vi "GetTerms4.vi"(0 "XRef":T11, 1 "State In":T10) -> (14 "Terms":T2, 15 "Fatal Error Out":T1)   [LabVIEW 2015, in "Set Object Parameters.xnode"]
uses:
  Set Object Parameters.xnode
  <vilib>/XNodeSupport/XNodeXNodeRef.ctl
  State.ctl
  <vilib>/XNodeSupport/XNodeTerm4Array.ctl
  <vilib>/XNodeSupport/XNodeTerm4.ctl
  <vilib>/XNodeSupport/XNodeString.ctl
  <vilib>/XNodeSupport/XNodeVariant.ctl
  <vilib>/XNodeSupport/XNodeRect32.ctl
  <vilib>/XNodeSupport/XNodeInt.ctl
  <vilib>/XNodeSupport/XNodeBool.ctl
  <vilib>/XNodeSupport/XNodeTermDirection.ctl
  <vilib>/XNodeSupport/XNodeErrorCluster.ctl
  JSON Object.lvclass
  JSON Datatype/JSON Null.lvclass
  JSON String/JSON String.lvclass
  JSON Numeric/JSON Numeric.lvclass
  JSON Boolean/JSON Boolean.lvclass
  JSON Array/JSON Array.lvclass
  dimensions.vi
  <vilib>/XNodeSupport/NI_XNodeSupport.lvlib
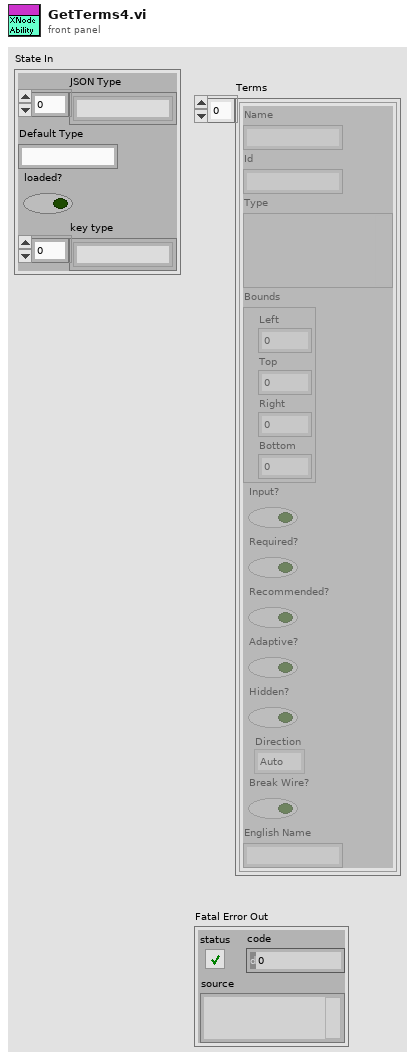
[diagram p1: front panel]
types:
  T1 = typedef "NI_XNodeSupport.lvlib/XNodeErrorCluster.ctl" = errorcluster
  T2 = typedef "NI_XNodeSupport.lvlib/XNodeTerm4Array.ctl" = T3[]
  T3 = typedef "NI_XNodeSupport.lvlib/XNodeTerm4.ctl" = cluster{"Name":T4, "Id":T4, "Type":T5, "Bounds":T6, "Input?":T8, "Required?":T8, "Recommended?":T8, "Adaptive?":T8, "Hidden?":T8, "Direction":T9, "Break Wire?":T8, "English Name":T4}
  T4 = typedef "NI_XNodeSupport.lvlib/XNodeString.ctl" = string
  T5 = typedef "NI_XNodeSupport.lvlib/XNodeVariant.ctl" = variant
  T6 = typedef "NI_XNodeSupport.lvlib/XNodeRect32.ctl" = cluster{"Left":T7, "Top":T7, "Right":T7, "Bottom":T7}
  T7 = typedef "NI_XNodeSupport.lvlib/XNodeInt.ctl" = i32
  T8 = typedef "NI_XNodeSupport.lvlib/XNodeBool.ctl" = bool
  T9 = typedef "NI_XNodeSupport.lvlib/XNodeTermDirection.ctl" = enum32{"Auto", "Up", "Down", "Left", "Right", "Center"}
  T10 = typedef "Set Object Parameters.xnode/State.ctl" = cluster{"JSON Type":string[], "Default Type":string, "loaded?":bool, "key type":string[]}
  T11 = typedef "NI_XNodeSupport.lvlib/XNodeXNodeRef.ctl" = refnum<vi>
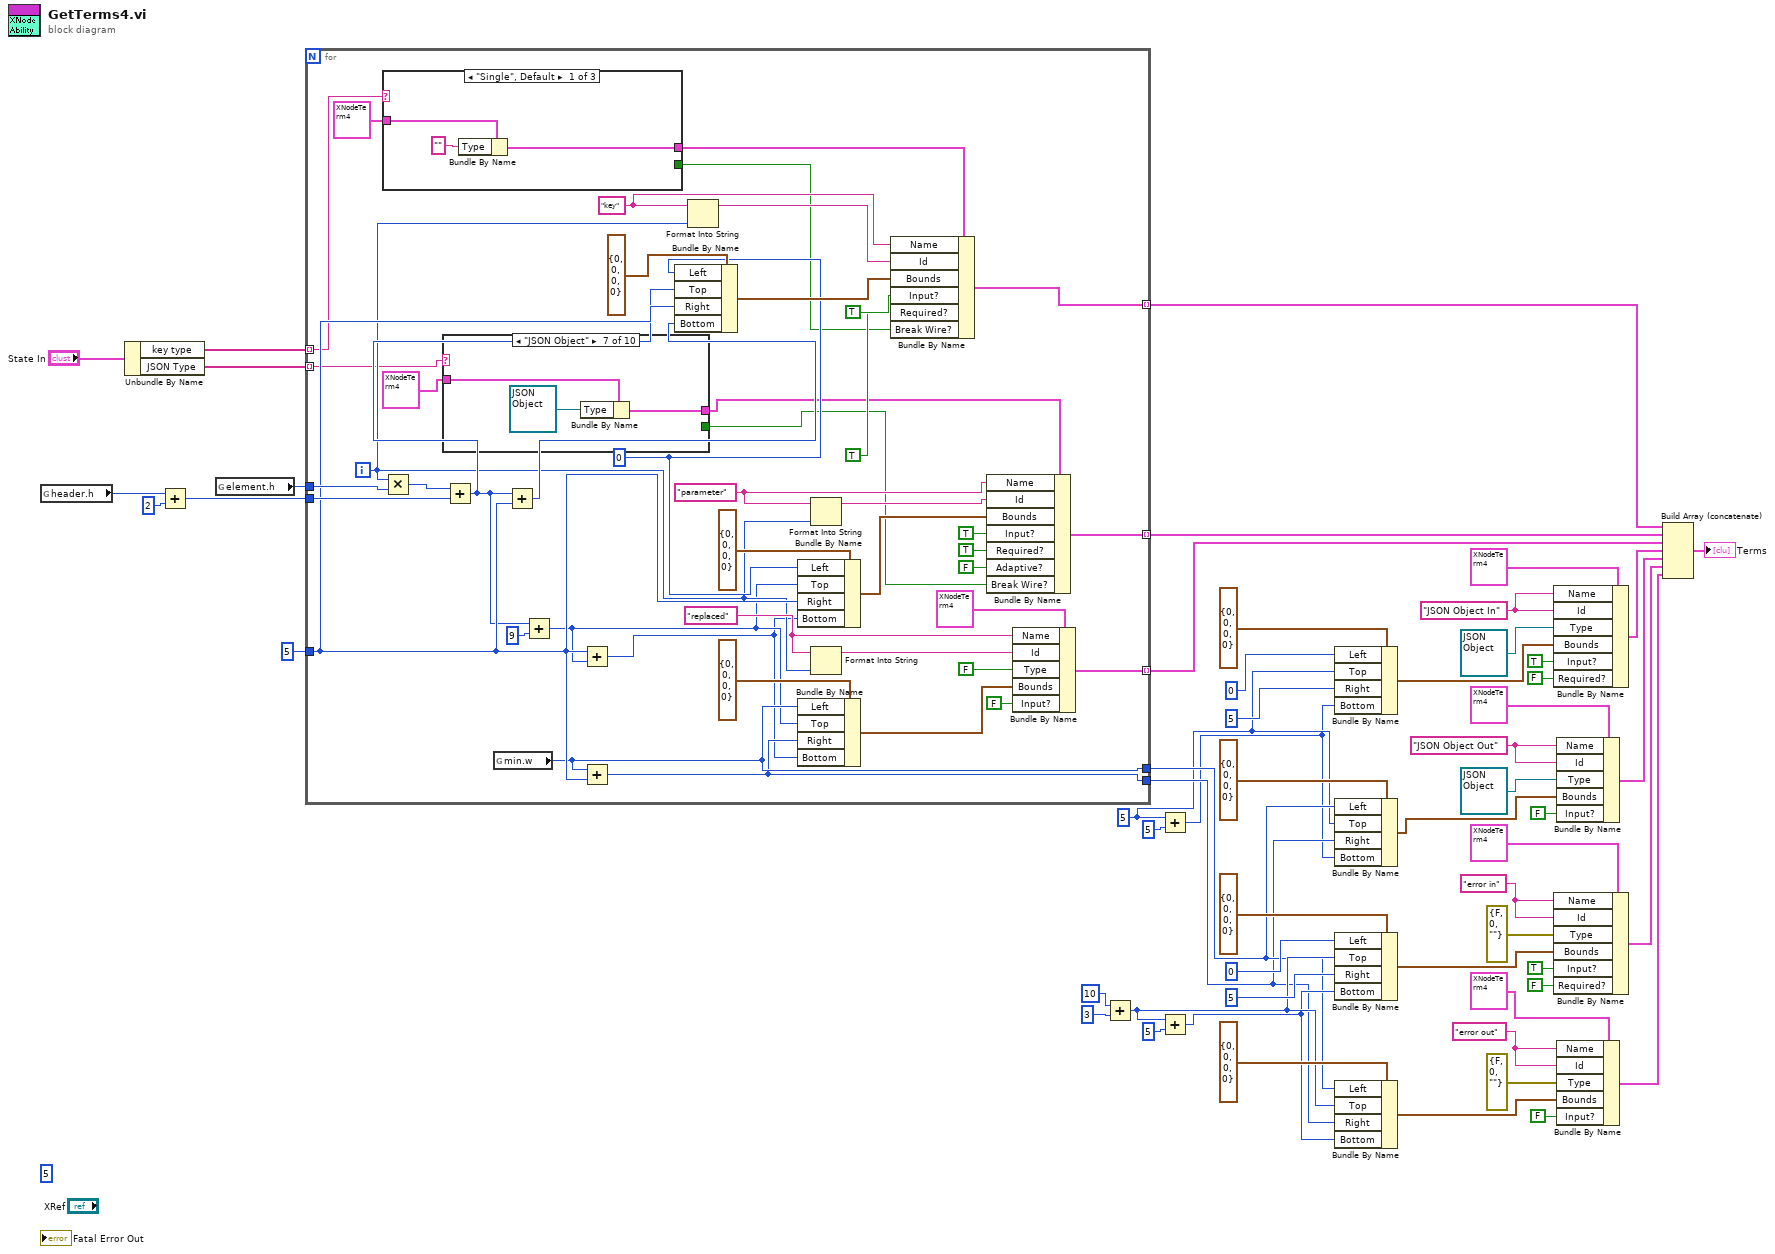
[diagram p0: block diagram]
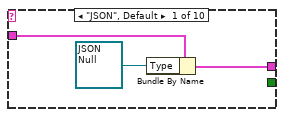
[diagram p2: hidden frame]
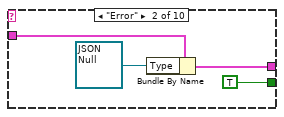
[diagram p3: hidden frame]
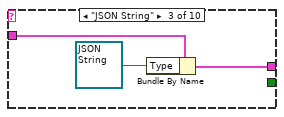
[diagram p4: hidden frame]
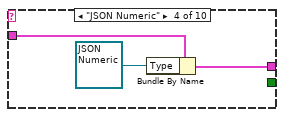
[diagram p5: hidden frame]
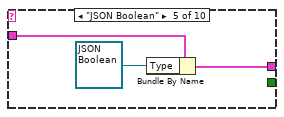
[diagram p6: hidden frame]
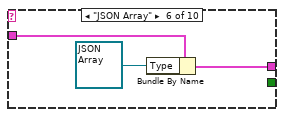
[diagram p7: hidden frame]
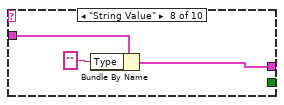
[diagram p8: hidden frame]
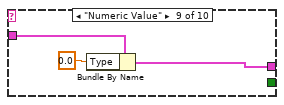
[diagram p9: hidden frame]
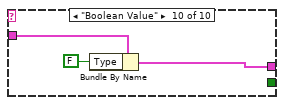
[diagram p10: hidden frame]
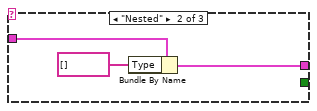
[diagram p11: hidden frame]
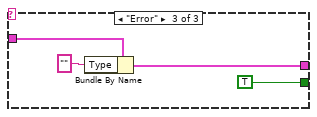
[diagram p12: hidden frame]
diagram:
  (unwired) T7 5 ("Right")
  w14 = T4 "JSON Object Out" ("Name")
  w22 = T4 "error out" ("Name")
  w33 = T4 "error in" ("Name")
  w6 = T7 5 ("Top")
  w45 = T4 "JSON Object In" ("Name")
  n1 = global read "dimensions.vi" "header.h"() -> (w53:i16)
  n2 = Unbundle By Name("State In") -> ("key type"=w1:string[], "JSON Type"=w4:string[])
  n3 = Add(x=w53, y=2) -> (x+y=w51:i32)
  n4 = global read "dimensions.vi" "element.h"() -> (w55:i16)
  n5 = for {
    tunnel: w55 -> [w97]
    tunnel: w51 -> [w94]
    tunnel: T7 5 ("Right") -> [w84]
    tunnel: [w89] -> w39 mode=indexing
    tunnel: [w88] -> w38 mode=indexing
    tunnel: w4 -> [w60] mode=indexing
    tunnel: [w69] -> w8
    tunnel: [w68] -> w7
    tunnel: [w76] -> w2 mode=indexing
    tunnel: w1 -> [w64] mode=indexing
    i -> [w71]
    w72 = "replaced" ("initial string")
    w73 = "parameter" ("initial string")
    w85 = T7 0 ("Left")
    w75 = "key" ("initial string")
    n6 = case shown="\"Single\", Default" w64 {
      tunnel: T3 {"Name"="", "Id"="", "Type"=variant, "Bounds"={"Left"=0, "Top"=0, "Right"=0, "Bottom"=0}, "Input?"=FALSE, "Required?"=FALSE, "Recommended?"=FALSE, "Adaptive?"=FALSE, "Hidden?"=FALSE, "Direction"=enum."Auto", "Break Wire?"=FALSE, "English Name"=""} ("Term 4") -> [w133 w136 w140]
      tunnel: [w132 w135 w139] -> w62
      tunnel: [_ _ T8 TRUE ("Break Wire?")] -> w61
      frame "Single", Default {
        n7 = Bundle By Name(cluster=w133, "Type"="" ("initial string")) -> (w132:T3)
      }
      frame "Nested" {
        n8 = Bundle By Name(cluster=w136, "Type"=string[] [] ("initial string")) -> (w135:T3)
      }
      frame "Error" {
        n9 = Bundle By Name(cluster=w140, "Type"="" ("initial string")) -> (w139:T3)
      }
    }
    n10 = Multiply(x=w71, y=w97) -> (x*y=w95:i32)
    n11 = case shown="\"JSON Object\"" w60 {
      tunnel: T3 {"Name"="", "Id"="", "Type"=variant, "Bounds"={"Left"=0, "Top"=0, "Right"=0, "Bottom"=0}, "Input?"=FALSE, "Required?"=FALSE, "Recommended?"=FALSE, "Adaptive?"=FALSE, "Hidden?"=FALSE, "Direction"=enum."Auto", "Break Wire?"=FALSE, "English Name"=""} ("Term 4") -> [w103 w107 w110 w113 w116 w119 w122 w125 w128 w131]
      tunnel: [w101 w105 w108 w111 w114 w117 w120 w124 w127 w130] -> w58
      tunnel: [_ T8 TRUE ("Break Wire?") _ _ _ _ _ _ _ _] -> w57
      frame "JSON", Default {
        n12 = Bundle By Name(cluster=w103, "Type"=refnum<class "JSON Null.lvclass"> refnum ("LVJSON.lvlib:JSON Null.lvclass")) -> (w101:T3)
      }
      frame "Error" {
        n13 = Bundle By Name(cluster=w107, "Type"=refnum<class "JSON Null.lvclass"> refnum ("LVJSON.lvlib:JSON Null.lvclass")) -> (w105:T3)
      }
      frame "JSON String" {
        n14 = Bundle By Name(cluster=w110, "Type"=refnum<class "JSON String.lvclass"> refnum ("LVJSON.lvlib:JSON String.lvclass")) -> (w108:T3)
      }
      frame "JSON Numeric" {
        n15 = Bundle By Name(cluster=w113, "Type"=refnum<class "JSON Numeric.lvclass"> refnum ("LVJSON.lvlib:JSON Numeric.lvclass")) -> (w111:T3)
      }
      frame "JSON Boolean" {
        n16 = Bundle By Name(cluster=w116, "Type"=refnum<class "JSON Boolean.lvclass"> refnum ("LVJSON.lvlib:JSON Boolean.lvclass")) -> (w114:T3)
      }
      frame "JSON Array" {
        n17 = Bundle By Name(cluster=w119, "Type"=refnum<class "JSON Array.lvclass"> refnum ("LVJSON.lvlib:JSON Array.lvclass")) -> (w117:T3)
      }
      frame "JSON Object" {
        n18 = Bundle By Name(cluster=w122, "Type"=refnum<class "JSON Object.lvclass"> refnum ("LVJSON.lvlib:JSON Object.lvclass")) -> (w120:T3)
      }
      frame "String Value" {
        n19 = Bundle By Name(cluster=w125, "Type"="" ("initial string")) -> (w124:T3)
      }
      frame "Numeric Value" {
        n20 = Bundle By Name(cluster=w128, "Type"=0.0) -> (w127:T3)
      }
      frame "Boolean Value" {
        n21 = Bundle By Name(cluster=w131, "Type"=FALSE) -> (w130:T3)
      }
    }
    n22 = Add(x=w95, y=w94) -> (x+y=w82:i32)
    n23 = global read "dimensions.vi" "min.w"() -> (w69:i32)
    n24 = Add(x=w82, y=w84) -> (x+y=w83:T7)
    n25 = Add(x=w82, y=9) -> (x+y=w67:i32)
    n26 = Add(x=w84, y=w67) -> (x+y=w66:T7)
    n27 = Add(x=w69, y=w84) -> (x+y=w68:T7)
    n28 = Bundle By Name(cluster=T6 {"Left"=0, "Top"=0, "Right"=0, "Bottom"=0} ("Bounds"), "Left"=w85, "Top"=w82, "Right"=w84, "Bottom"=w83) -> (w96:T6)
    n29 = Format Into String(initial string=w75, w71) -> (resulting string=w74:string)  [unwired: 2 in, 1 out]
    n30 = Bundle By Name(cluster=T6 {"Left"=0, "Top"=0, "Right"=0, "Bottom"=0} ("Bounds"), "Left"=w85, "Top"=w67, "Right"=w84, "Bottom"=w66) -> (w93:T6)
    n31 = Bundle By Name(cluster=T6 {"Left"=0, "Top"=0, "Right"=0, "Bottom"=0} ("Bounds"), "Left"=w69, "Top"=w67, "Right"=w68, "Bottom"=w66) -> (w80:T6)
    n32 = Format Into String(initial string=w73, w71) -> (resulting string=w65:string)  [unwired: 2 in, 1 out]
    n33 = Format Into String(initial string=w72, w71) -> (resulting string=w70:string)  [unwired: 2 in, 1 out]
    n34 = Bundle By Name(cluster=w62, "Name"=w75, "Id"=w74, "Bounds"=w96, "Input?"=T8 TRUE, "Required?"=T8 TRUE, "Break Wire?"=w61) -> (w88:T3)
    n35 = Bundle By Name(cluster=w58, "Name"=w73, "Id"=w65, "Bounds"=w93, "Input?"=T8 TRUE, "Required?"=T8 TRUE, "Adaptive?"=T8 FALSE, "Break Wire?"=w57) -> (w89:T3)
    n36 = Bundle By Name(cluster=T3 {"Name"="", "Id"="", "Type"=variant, "Bounds"={"Left"=0, "Top"=0, "Right"=0, "Bottom"=0}, "Input?"=FALSE, "Required?"=FALSE, "Recommended?"=FALSE, "Adaptive?"=FALSE, "Hidden?"=FALSE, "Direction"=enum."Auto", "Break Wire?"=FALSE, "English Name"=""} ("Term 4"), "Name"=w72, "Id"=w70, "Type"=FALSE, "Bounds"=w80, "Input?"=T8 FALSE) -> (w76:T3)
  }
  n37 = Add(x=T7 10, y=T7 3) -> (x+y=w19:T7)
  n38 = Add(x=w6, y=T7 5) -> (x+y=w5:T7)
  n39 = Add(x=w19, y=T7 5) -> (x+y=w18:T7)
  n40 = Bundle By Name(cluster=T6 {"Left"=0, "Top"=0, "Right"=0, "Bottom"=0} ("Bounds"), "Left"=T7 0, "Top"=w6, "Right"=T7 5, "Bottom"=w5) -> (w46:T6)
  n41 = Bundle By Name(cluster=T6 {"Left"=0, "Top"=0, "Right"=0, "Bottom"=0} ("Bounds"), "Left"=w8, "Top"=w6, "Right"=w7, "Bottom"=w5) -> (w13:T6)
  n42 = Bundle By Name(cluster=T6 {"Left"=0, "Top"=0, "Right"=0, "Bottom"=0} ("Bounds"), "Left"=T7 0, "Top"=w19, "Right"=T7 5, "Bottom"=w18) -> (w32:T6)
  n43 = Bundle By Name(cluster=T6 {"Left"=0, "Top"=0, "Right"=0, "Bottom"=0} ("Bounds"), "Left"=w8, "Top"=w19, "Right"=w7, "Bottom"=w18) -> (w23:T6)
  n44 = Bundle By Name(cluster=T3 {"Name"="", "Id"="", "Type"=variant, "Bounds"={"Left"=0, "Top"=0, "Right"=0, "Bottom"=0}, "Input?"=FALSE, "Required?"=FALSE, "Recommended?"=FALSE, "Adaptive?"=FALSE, "Hidden?"=FALSE, "Direction"=enum."Auto", "Break Wire?"=FALSE, "English Name"=""} ("Term 4"), "Name"=w45, "Id"=w45, "Type"=refnum<class "JSON Object.lvclass"> refnum ("LVJSON.lvlib:JSON Object.lvclass"), "Bounds"=w46, "Input?"=T8 TRUE, "Required?"=T8 FALSE) -> (w41:T3)
  n45 = Bundle By Name(cluster=T3 {"Name"="", "Id"="", "Type"=variant, "Bounds"={"Left"=0, "Top"=0, "Right"=0, "Bottom"=0}, "Input?"=FALSE, "Required?"=FALSE, "Recommended?"=FALSE, "Adaptive?"=FALSE, "Hidden?"=FALSE, "Direction"=enum."Auto", "Break Wire?"=FALSE, "English Name"=""} ("Term 4"), "Name"=w33, "Id"=w33, "Type"=errorcluster {"status"=FALSE, "code"=0, "source"=""} ("error constant"), "Bounds"=w32, "Input?"=T8 TRUE, "Required?"=T8 FALSE) -> (w16:T3)
  n46 = Bundle By Name(cluster=T3 {"Name"="", "Id"="", "Type"=variant, "Bounds"={"Left"=0, "Top"=0, "Right"=0, "Bottom"=0}, "Input?"=FALSE, "Required?"=FALSE, "Recommended?"=FALSE, "Adaptive?"=FALSE, "Hidden?"=FALSE, "Direction"=enum."Auto", "Break Wire?"=FALSE, "English Name"=""} ("Term 4"), "Name"=w14, "Id"=w14, "Type"=refnum<class "JSON Object.lvclass"> refnum ("LVJSON.lvlib:JSON Object.lvclass"), "Bounds"=w13, "Input?"=T8 FALSE) -> (w9:T3)
  n47 = Bundle By Name(cluster=T3 {"Name"="", "Id"="", "Type"=variant, "Bounds"={"Left"=0, "Top"=0, "Right"=0, "Bottom"=0}, "Input?"=FALSE, "Required?"=FALSE, "Recommended?"=FALSE, "Adaptive?"=FALSE, "Hidden?"=FALSE, "Direction"=enum."Auto", "Break Wire?"=FALSE, "English Name"=""} ("Term 4"), "Name"=w22, "Id"=w22, "Type"=errorcluster {"status"=FALSE, "code"=0, "source"=""} ("error constant"), "Bounds"=w23, "Input?"=T8 FALSE) -> (w20:T3)
  n48 = Build Array (concatenate)(w38, w39, w2, w41, w9, w16, w20) -> (→"Terms":T3[])
